vi "sub_measure_distance.vi"(10 "pt 2":cluster{"x":dbl, "y":dbl}, 11 "pt 1":cluster{"x":dbl, "y":dbl}) -> (3 "distance":dbl)   [LabVIEW 2019]
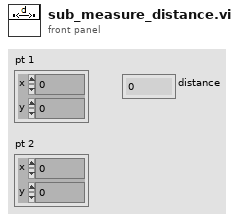
[diagram p1: front panel]
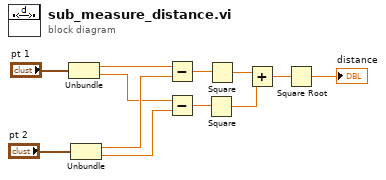
[diagram p0: block diagram]
diagram:
  n1 = Unbundle("pt 1") -> ("x"=w4:dbl, "y"=w2:dbl)
  n2 = Unbundle("pt 2") -> ("x"=w3:dbl, "y"=w1:dbl)
  n3 = Subtract(x=w4, y=w3) -> (x-y=w8:dbl)
  n4 = Subtract(x=w2, y=w1) -> (x-y=w6:dbl)
  n5 = Square(x=w6) -> (x^2=w7:dbl)
  n6 = Square(x=w8) -> (x^2=w9:dbl)
  n7 = Add(x=w9, y=w7) -> (x+y=w10:dbl)
  n8 = Square Root(x=w10) -> (sqrt(x)=→"distance":dbl)
